vi "Save ROI.vi"(10 "File path":path, 11 "ROI":T1) -> ()   [LabVIEW 2016]
uses:
  <vilib>/vision/NI_Vision_Development_Module.lvlib
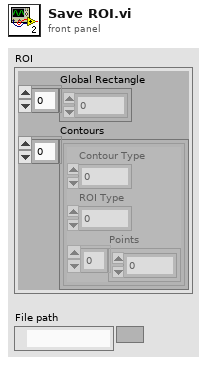
[diagram p1: front panel]
types:
  T1 = cluster{"Global Rectangle":i32[], "Contours":cluster{"Contour Type":u32, "ROI Type":u32, "Points":i32[]}[]}
  T2 = typedef "IMAQ Image.ctl" = refnum<image>
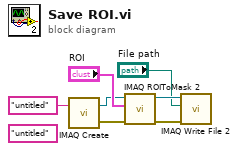
[diagram p0: block diagram]
diagram:
  (unwired) "untitled" ("Image Name")
  n1 = call "IMAQ Create"("Image Name"="untitled") -> ("New Image"=w3:T2, "error out"=w6:errorcluster)  [unwired: 4 in]
  n2 = call "IMAQ ROIToMask 2"("error in (no error)"=w6, "ROI Descriptor"="ROI", "Image"=w3) -> ("error out"=w7:errorcluster, "Image Out"=w4:T2)  [unwired: 6 in, 1 out]
  n3 = call-poly "IMAQ Write File 2"("error in (no error)"=w7, "File Path"="File path", "Image"=w4) -> ()  [unwired: 7 in, 2 out]
